vi "mod_Generate analytic signal.vi"(0 "m(t)":dbl[](array[numeric]), 5 "filter taps":cdb[](array[numeric]), 11 "error in (no error)":errorcluster, 13 "reset? (T)":bool=TRUE) -> (4 "analytic signal":cdb[](array[numeric]), 15 "error out":errorcluster)   [LabVIEW 2020, in "niAMT.lvlib"]
uses:
  <vilib>/addons/Modulation/niAMT.lvlib
  <vilib>/Analysis/3filter.llb/IIR Filter (DBL).vi
  <vilib>/Analysis/NI_AALBase.lvlib
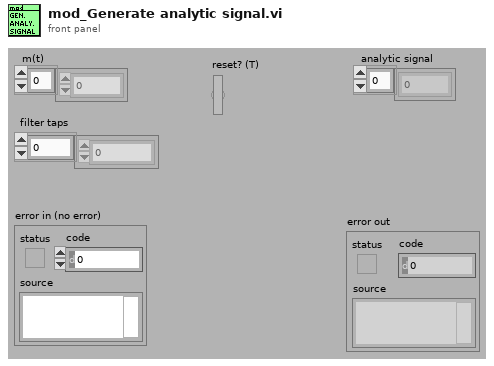
[diagram p1: front panel]
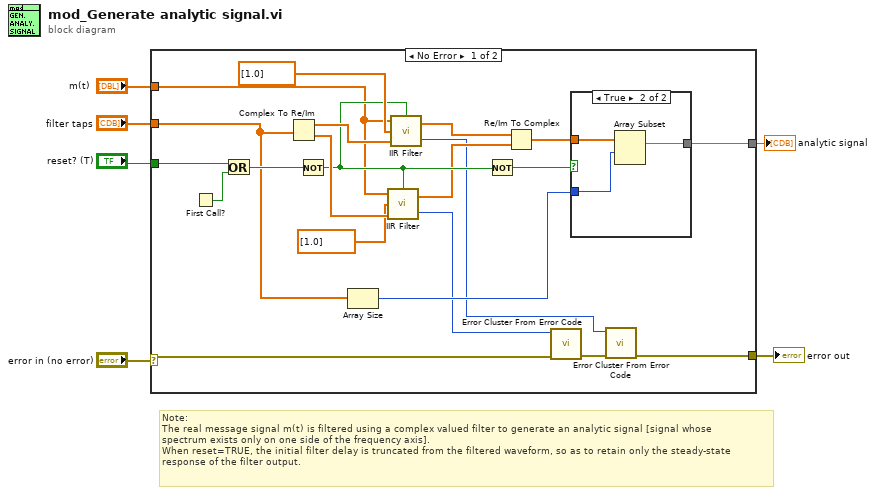
[diagram p0: block diagram]
diagram:
  # "Note:\nThe real message signal m(t) is filtered using a complex valued filter to generate an analytic signal [signal whose\nspectrum exists only on one side of the frequency axis].\nWhen reset=TRUE, the initial filter delay is truncated from the filtered waveform, so as to retain only the steady-state\nresponse of the filter output."
  n1 = case shown="No Error" "error in (no error)" {
    selector: "error in (no error)" -> [w11 w32]
    tunnel: [w7 w32] -> w5
    tunnel: "m(t)" -> [w15 _]
    tunnel: "filter taps" -> [w14 _]
    tunnel: "reset? (T)" -> [w13 _]
    tunnel: [w12 _] -> w1
    frame No Error {
      n2 = First Call?() -> (First Call?: T/F=w27:bool)
      n3 = Or(x=w13, y=w27) -> (x .or. y?=w26:bool)
      n4 = Complex To Re/Im(x + iy=w14) -> (x=w25:dbl[], y=w24:dbl[])
      n5 = Not(x=w26) -> (.not. x?=w21:bool)
      n6 = Array Size(array=w14) -> (size(s)=w16:i32)
      n7 = call-poly <vilib>:"IIR Filter.vi"("init/cont (init:F)"=w21, "Forward Coefficients"=w24, "Reverse Coefficients"=dbl[] [1.0], "X"=w15) -> ("error"=w10:i32, "Filtered X"=w18:dbl[])
      n8 = call-poly <vilib>:"IIR Filter.vi"("init/cont (init:F)"=w21, "Forward Coefficients"=w25, "Reverse Coefficients"=dbl[] [1.0], "X"=w15) -> ("error"=w9:i32, "Filtered X"=w19:dbl[])
      n9 = Not(x=w21) -> (.not. x?=w20:bool)
      n10 = Re/Im To Complex(1:w18, 2:w19) -> (0:w17:cdb[])
      n11 = call <vilib>:"Error Cluster From Error Code.vi"("error in (no error)"=w11, "error code (0)"=w10) -> ("error out"=w8:errorcluster)  [unwired: 1 in, 6 out]
      n12 = case shown="True" w20 {
        tunnel: w17 -> [w28 w31]
        tunnel: [w28 w30] -> w12
        tunnel: w16 -> [_ w29]
        frame False {
        }
        frame True {
          n13 = Array Subset(array=w31, index=w29) -> (w30:cdb[])  [unwired: 1 in]
        }
      }
      n14 = call <vilib>:"Error Cluster From Error Code.vi"("error in (no error)"=w8, "error code (0)"=w9) -> ("error out"=w7:errorcluster)  [unwired: 1 in, 6 out]
    }
    frame Error {
    }
  }
  "error out" <- w5
  "analytic signal" <- w1
